vi "Mass Compile Source.vi"(8 "error in (no error)":errorcluster, 11 "Configuration in":T1) -> (0 "error out":errorcluster, 3 "Configuration out":T1)   [LabVIEW 2011, in "LVH-Build-Tools.lvlib"]
uses:
  LVH-Build-Tools.lvlib
  Type Defs/Configuration.ctl
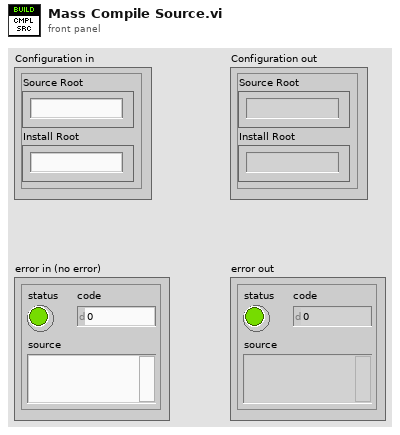
[diagram p1: front panel]
types:
  T1 = typedef "LVH-Build-Tools.lvlib/Configuration.ctl" = cluster{"Source Root":string, "Install Root":string, "Components":string[], "Ignore":string[]}
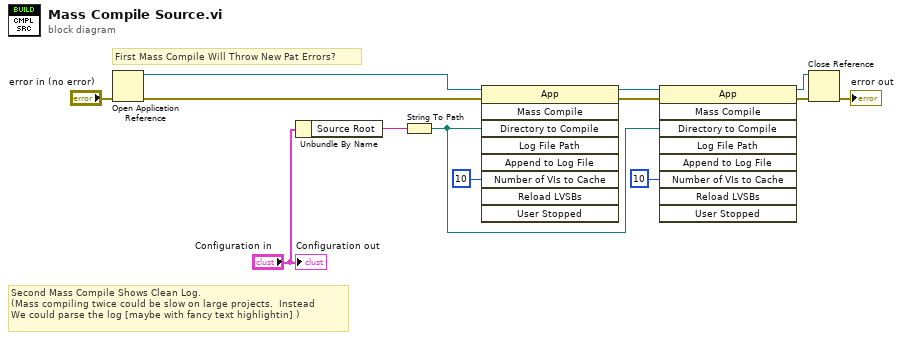
[diagram p0: block diagram]
diagram:
  # "Second Mass Compile Shows Clean Log.\n(Mass compiling twice could be slow on large projects.  Instead \nWe could parse the log [maybe with fancy text highlightin] )"
  # "First Mass Compile Will Throw New Pat Errors?"
  n1 = Open Application Reference(8:"error in (no error)") -> (0:w5:errorcluster, 3:w6:refnum<vi>)  [unwired: 3 in]
  n2 = Unbundle By Name("Configuration in") -> ("Source Root"=w4:string)
  n3 = String To Path(string=w4) -> (path=w11:path)
  n4 = invoke class="App" method="Mass Compile"(reference=w6, error in=w5, "Directory to Compile"=w11, "Number of VIs to Cache"=u32 10) -> (reference out=w12:refnum<vi>, error out=w13:errorcluster)  [unwired: 5 in, 7 out]
  n5 = invoke class="App" method="Mass Compile"(reference=w12, error in=w13, "Directory to Compile"=w11, "Number of VIs to Cache"=u32 10) -> (reference out=w9:refnum<vi>, error out=w10:errorcluster)  [unwired: 5 in, 7 out]
  n6 = Close Reference(reference=w9, error in (no error)=w10) -> (error out=→"error out":errorcluster)
  "Configuration out" <- "Configuration in"
